vi "Publish (Control Packet).vi"(6 "timeout (1000ms)":i32=1000, 8 "error in (no error)":errorcluster, 10 "PUBLISH":refnum<class "PUBLISH.lvclass">, 11 "Client in":refnum<class "Client.lvclass">) -> (0 "error out":errorcluster, 2 "Published":bool, 3 "Client out":refnum<class "Client.lvclass">)   [LabVIEW 2013, in "MQTT Client.lvlib" / "Client.lvclass"]
uses:
  Client.lvclass
  <vilib>/LabVIEW Open Source Project/MQTT Control Packets/Control Packets/PUBLISH/PUBLISH.lvclass
  <vilib>/LabVIEW Open Source Project/MQTT Control Packets/Control Packets/PUBCOMP/PUBCOMP.lvclass
  <vilib>/LabVIEW Open Source Project/MQTT Control Packets/Control Packets/PUBREC/PUBREC.lvclass
  <vilib>/LabVIEW Open Source Project/MQTT Control Packets/Control Packets/ControlPacket/ControlPacket.lvclass/ControlPacket.ctl
  <vilib>/LabVIEW Open Source Project/MQTT Control Packets/Control Packets/PUBACK/PUBACK.lvclass
  <vilib>/LabVIEW Open Source Project/MQTT Control Packets/Control Packets/ControlPacket/ControlPacket.lvclass
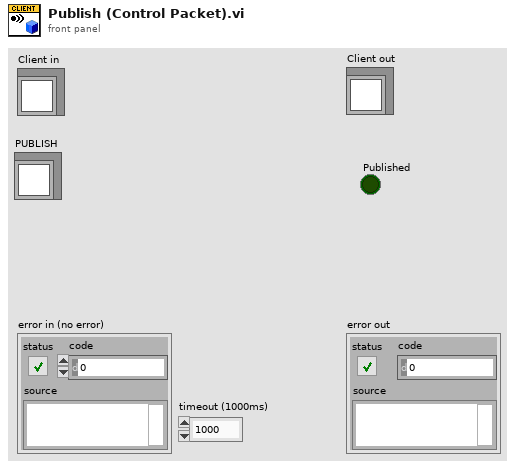
[diagram p1: front panel]
types:
  T1 = typedef "MQTT_Control_Packets.lvlib/ControlPacket.lvclass/QualityOfService -- enum.ctl" = enum16{"0 (At Most Once)", "1 (At Least Once)", "2 (Exactly Once)"}
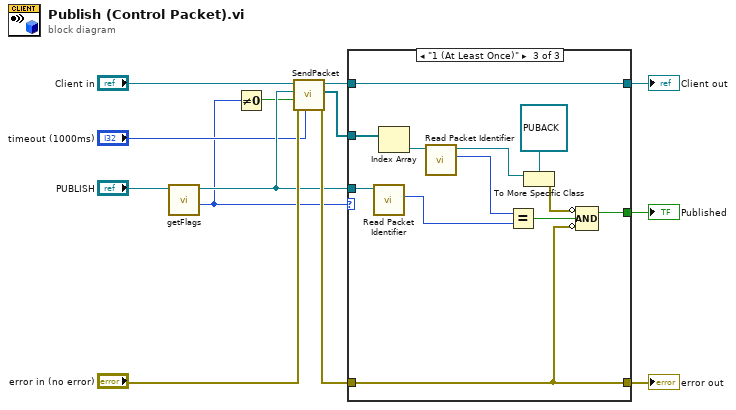
[diagram p0: block diagram]
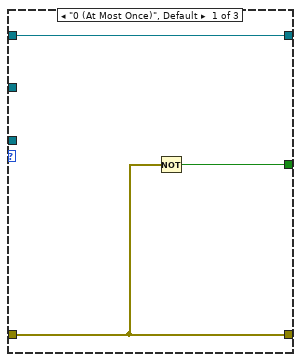
[diagram p2: hidden frame]
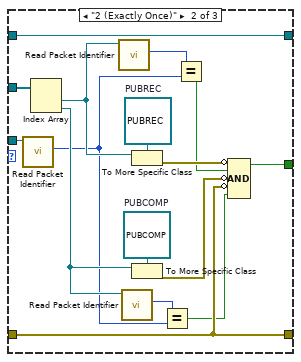
[diagram p3: hidden frame]
diagram:
  n1 = call-dynamic "getFlags.vi"("PUBLISH in"="PUBLISH") -> ("QoS"=w1:T1, "PUBLISH out"=w5:refnum<class "PUBLISH.lvclass">)  [unwired: 7 in, 2 out]
  n2 = Not Equal To 0?(x=w1) -> (x != 0?=w3:bool)
  n3 = call "SendPacket.vi"("timeout (1000ms)"="timeout (1000ms)", "error in (no error)"="error in (no error)", "Wait for ack? (T)"=w3, "ControlPacket"=w5, "Client in"="Client in") -> ("error out"=w9:errorcluster, "Response"=w7:refnum<class "ControlPacket.lvclass">[], "Client out"=w11:refnum<class "Client.lvclass">)  [unwired: 4 in]
  n4 = case shown="\"1 (At Least Once)\"" w1 {
    tunnel: w7 -> [_ w32 w44]
    tunnel: [w16 w26 w42] -> w8
    tunnel: w9 -> [w16 w26 w42]
    tunnel: [w15 w27 w38] -> w10
    tunnel: w11 -> [w14 w23 w43]
    tunnel: [w14 w23 w43] -> w12
    tunnel: w5 -> [_ w18 w37]
    frame "0 (At Most Once)", Default {
      n5 = Not(x=w16) -> (.not. x?=w15:bool)
    }
    frame "2 (Exactly Once)" {
      w31 = refnum<class "PUBREC.lvclass"> refnum  # PUBREC
      w30 = refnum<class "PUBCOMP.lvclass"> refnum  # PUBCOMP
      n6 = call <vilib>:"Read Packet Identifier.vi"("ControlPacket in"=w18) -> ("Packet Identifier"=w17:u16)  [unwired: 9 in, 1 out]
      n7 = Index Array(array=w32) -> (element #1=w21:refnum<class "ControlPacket.lvclass">, element #2=w20:refnum<class "ControlPacket.lvclass">)  [unwired: 2 in]
      n8 = call <vilib>:"Read Packet Identifier.vi"("ControlPacket in"=w21) -> ("Packet Identifier"=w22:u16)  [unwired: 9 in, 1 out]
      n9 = call <vilib>:"Read Packet Identifier.vi"("ControlPacket in"=w20) -> ("Packet Identifier"=w25:u16)  [unwired: 9 in, 1 out]
      n10 = To More Specific Class(target class=w31, reference=w21) -> (error out=w29:errorcluster)  [unwired: 1 in, 1 out]
      n11 = To More Specific Class(target class=w30, reference=w20) -> (error out=w28:errorcluster)  [unwired: 1 in, 1 out]
      n12 = Equal?(x=w25, y=w17) -> (x = y?=w24:bool)
      n13 = Equal?(x=w22, y=w17) -> (x = y?=w19:bool)
      n14 = Compound Arithmetic op=AND(invert w29, w19, invert w28, invert w26, w24) -> (w27:bool)
    }
    frame "1 (At Least Once)" {
      n15 = call <vilib>:"Read Packet Identifier.vi"("ControlPacket in"=w37) -> ("Packet Identifier"=w36:u16)  [unwired: 9 in, 1 out]
      n16 = Index Array(array=w44) -> (element=w39:refnum<class "ControlPacket.lvclass">)  [unwired: 1 in]
      n17 = call <vilib>:"Read Packet Identifier.vi"("ControlPacket in"=w39) -> ("Packet Identifier"=w41:u16, "ControlPacket out"=w33:refnum<class "ControlPacket.lvclass">)  [unwired: 9 in]
      n18 = Equal?(x=w41, y=w36) -> (x = y?=w40:bool)
      n19 = To More Specific Class(target class=refnum<class "PUBACK.lvclass"> refnum ("PUBACK out"), reference=w33) -> (error out=w34:errorcluster)  [unwired: 1 in, 1 out]
      n20 = Compound Arithmetic op=AND(invert w34, w40, invert w42) -> (w38:bool)
    }
  }
  "Client out" <- w12
  "Published" <- w10
  "error out" <- w8
